vi "趋势图对话框.vi"(8 "初始化":refnum<vi>, 9 "参数":string, 10 "Array输入":refnum<vi>, 11 "原点":T1 caption="点") -> ()   [LabVIEW 2016, in "多参数状态显示.xctl"]
uses:
  <vilib>/Utility/miscctls.llb/LVPointTypeDef.ctl
panel:
  out "波形图":dbl[](graph)
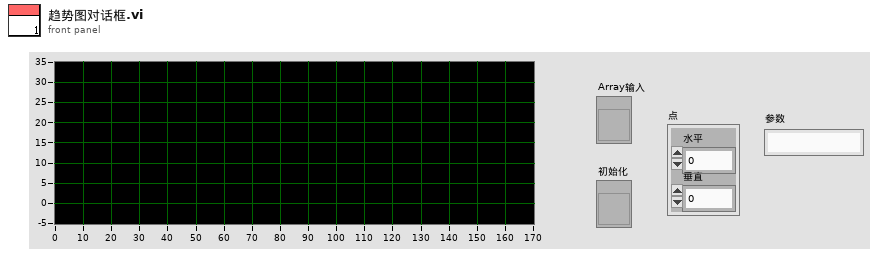
[diagram p1: front panel]
types:
  T1 = typedef "LVPointTypeDef.ctl" = cluster{"Horizontal":i16, "Vertical":i16}
  T2 = typedef "LVRectTypeDef.ctl" = cluster{"Left":i16, "Top":i16, "Right":i16, "Bottom":i16}
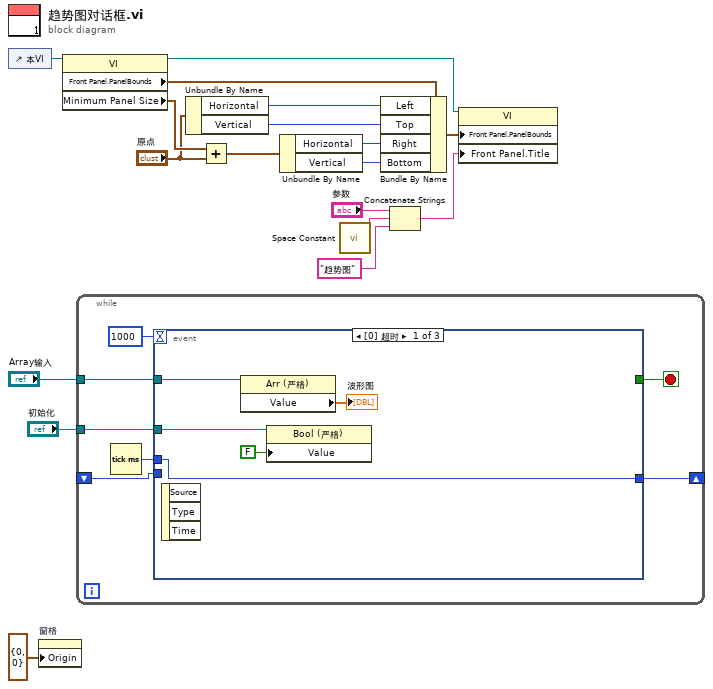
[diagram p0: block diagram]
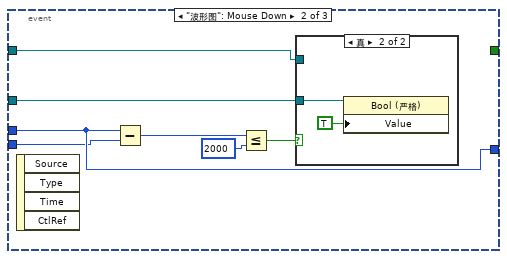
[diagram p2: hidden frame]
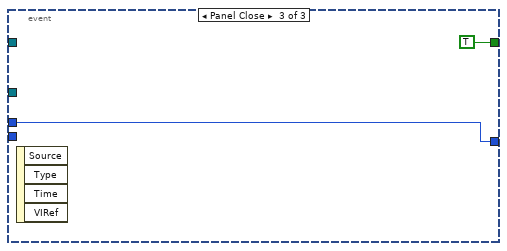
[diagram p4: hidden frame]
diagram:
  n1 = control-ref of="本VI"() -> (w17:refnum<vi>)
  n2 = property on="窗格" class="Pane"("Origin"=T1 {"Horizontal"=0, "Vertical"=0} ("原点")) -> ()  [unwired: 2 in, 2 out]
  n3 = property class="VI"(reference=w17) -> (reference out=w16:refnum<vi>, "Front Panel.PanelBounds"=w15:T2, "Minimum Panel Size"=w11:T1)  [unwired: 1 in, 1 out]
  n4 = while {
    tunnel: "Array输入" -> [w23]
    shift-right: [w21] -> _
    shift-left: _ -> [w20]
    tunnel: "初始化" -> [w19]
    stop <- w25 stop-if-true
    n5 = Tick Count (ms)() -> (millisecond timer value=w22:u32)
    n6 = event shown="[0] 超时" {
      selector: _ -> [_ _ _]
      dyn-events: _ -> [_ _ _]
      timeout: 1000 -> [_ _ _]
      tunnel: [_ _ TRUE] -> w25
      tunnel: w23 -> [w30 w32 _]
      tunnel: w22 -> [w28 w37 w40]
      tunnel: [w28 w37 w40] -> w21
      tunnel: w20 -> [_ w36 _]
      tunnel: w19 -> [w27 w31 _]
      event Timeout {
        n7 = event-data() -> ()  [unwired: 1 in, 3 out]
        n8 = property class="Arr (严格)"(reference=w30) -> ("Value"=→"波形图":dbl[])  [unwired: 1 in, 2 out]
        n9 = property class="Bool (严格)"(reference=w27, "Value"=FALSE ("值")) -> ()  [unwired: 1 in, 2 out]
      }
      event "波形图": Mouse Down {
        n10 = event-data() -> ()  [unwired: 1 in, 4 out]
        n11 = Subtract(x=w37, y=w36) -> (x-y=w35:u32)
        n12 = Less Or Equal?(x=w35, y=u32 2000) -> (x <= y?=w33:bool)
        n13 = case shown="真" w33 {
          tunnel: w32 -> [_ _]
          tunnel: w31 -> [_ w39]
          frame False {
          }
          frame True {
            n14 = property class="Bool (严格)"(reference=w39, "Value"=TRUE ("值")) -> ()  [unwired: 1 in, 2 out]
          }
        }
      }
      event Panel Close {
        n15 = event-data() -> ()  [unwired: 1 in, 4 out]
      }
    }
  }
  n16 = Unbundle By Name("原点") -> ("Horizontal"=w13:i16, "Vertical"=w12:i16)
  n17 = Add(x=w11, y="原点") -> (x+y=w9:T1)
  n18 = Unbundle By Name(w9) -> ("Horizontal"=w8:i16, "Vertical"=w7:i16)
  n19 = call <vilib>:"Space Constant.vi"() -> ("String"=w2:string)
  n20 = Bundle By Name(cluster=w15, "Left"=w13, "Top"=w12, "Right"=w8, "Bottom"=w7) -> (w14:T2)
  n21 = Concatenate Strings("参数", w2, "趋势图" ("字符串")) -> (w4:string)
  n22 = property class="VI"(reference=w16, "Front Panel.PanelBounds"=w14, "Front Panel.Title"=w4) -> ()  [unwired: 1 in, 2 out]
